vi "DataHandler Type.vi"(8 "error in (no error)":errorcluster, 11 "PublishDataHandler in":refnum<class "PublishDataHandler.lvclass">) -> (0 "error out":errorcluster, 2 "DataHandler Type":string, 3 "PublishDataHandler out":refnum<class "PublishDataHandler.lvclass">)   [LabVIEW 2020, in "VolatusDataProcessing.lvlib" / "PublishDataHandler.lvclass"]
uses:
  PublishDataHandler.lvclass
  PublishDataHandler.lvclass/PublishDataHandler.ctl
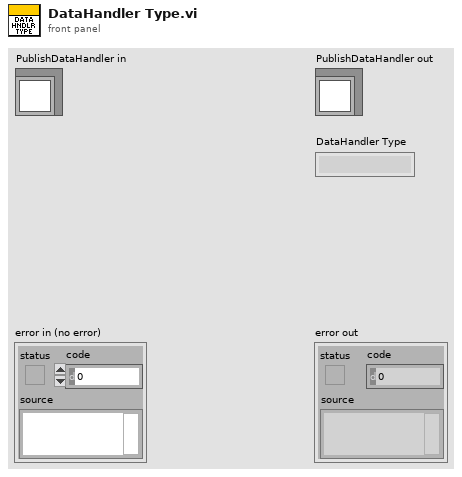
[diagram p1: front panel]
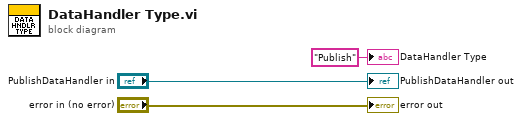
[diagram p0: block diagram]
diagram:
  "error out" <- "error in (no error)"
  "PublishDataHandler out" <- "PublishDataHandler in"
  "DataHandler Type" <- "Publish" ("DataHandler Type")
